vi "WriteSave2MarkdownWithImages.vi"(0 "Measurement type":T3(ring)=enum."Spectrum", 1 "Full Comment":string, 2 "Params Save":T2, 3 "Written Dataset Name":string, 4 "Log file":string caption="Status") -> (5 "Log file after":string)   [LabVIEW 2019]
uses:
  TypeDefs/AcqMode.ctl
panel:
  out "Experiment Name":string
  out "ExperimentTag":string
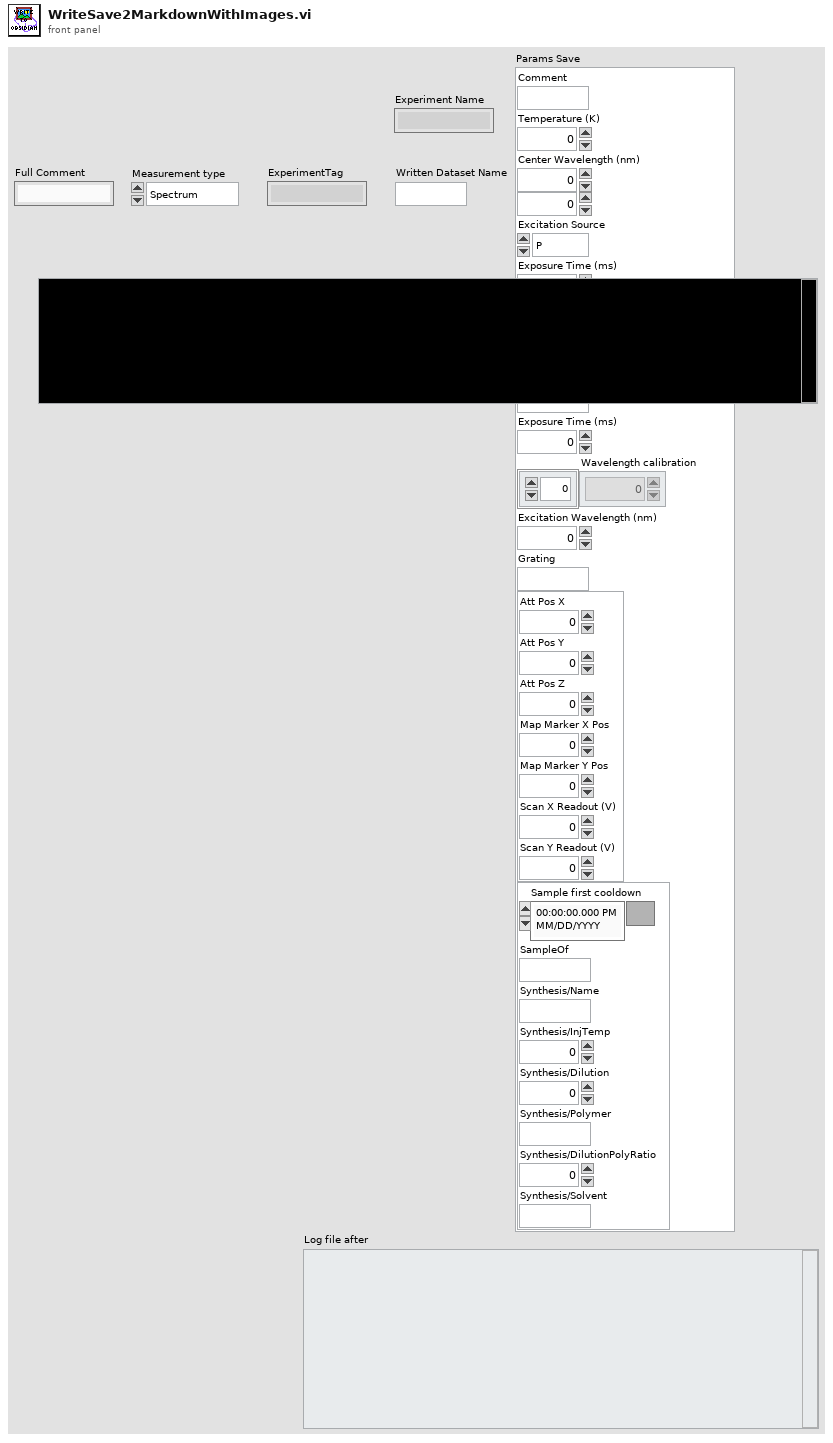
[diagram p1: front panel]
types:
  T1 = typedef "AcqMode.ctl" = enum16{"Image", "Spectrum", "APD 1", "APD 2", "APD 1+2"}
  T2 = cluster{"Comment":string, "Temperature (K)":dbl, "Center Wavelength (nm)":dbl, "Numeric":dbl, "Excitation Source":enum16{"P", "CW", "SK"}, "Exposure Time (ms)":dbl, "Experiment Name":string, "Acq Mode":T1, "Log file":string, "Exposure Time (ms)":dbl, "Wavelength calibration":dbl[], "Excitation Wavelength (nm)":dbl, "Grating":string, "Cluster":cluster{"Att Pos X":dbl, "Att Pos Y":dbl, "Att Pos Z":dbl, "Map Marker X Pos":i8, "Map Marker Y Pos":i8, "Scan X Readout (V)":dbl, "Scan Y Readout (V)":dbl}, "Cluster":cluster{"Sample first cooldown":timestamp, "SampleOf":string, "Synthesis/Name":string, "Synthesis/InjTemp":dbl, "Synthesis/Dilution":dbl, "Synthesis/Polymer":string, "Synthesis/DilutionPolyRatio":dbl, "Synthesis/Solvent":string}}
  T3 = enum16{"Time Trace", "Contrast", "XY Intensity Map", "Polarisation", "Spectrum", "Michelson", "fPow"}
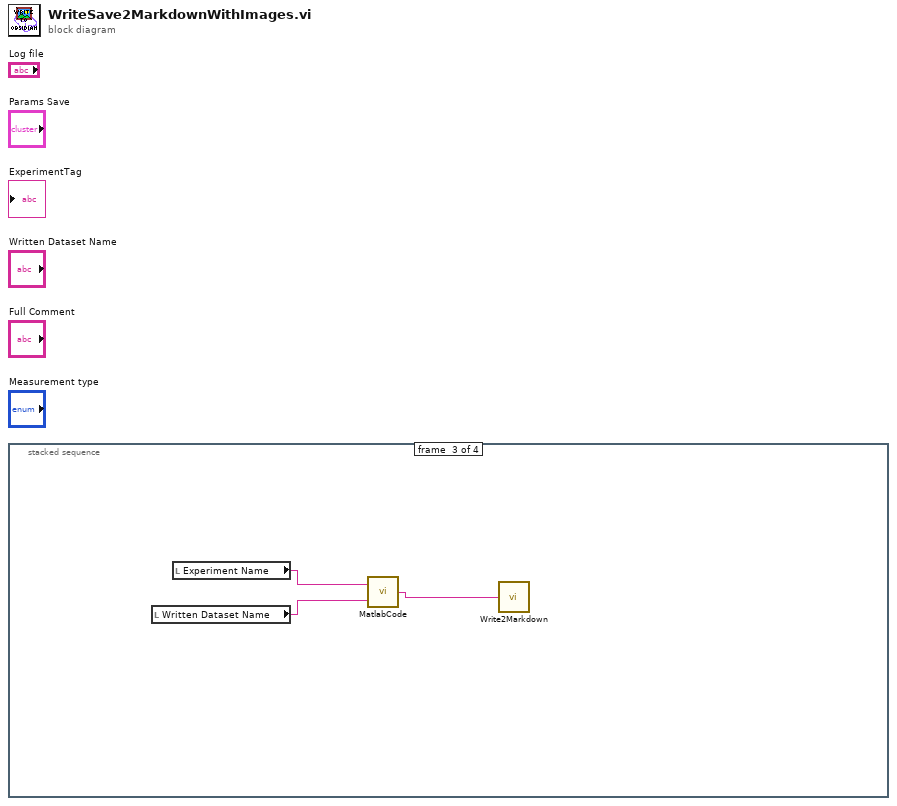
[diagram p0: block diagram]
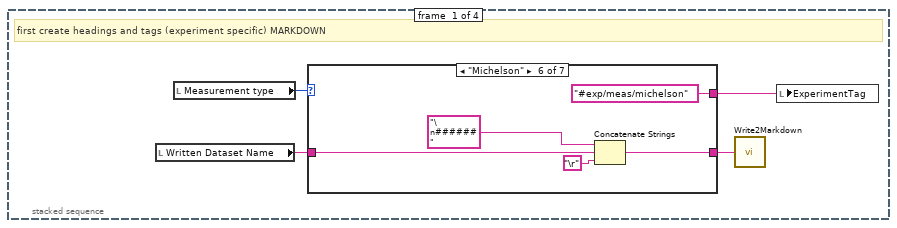
[diagram p2: hidden frame]
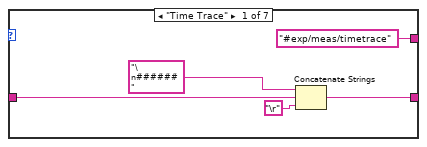
[diagram p3: hidden frame]
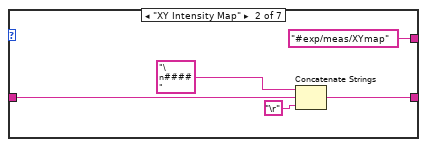
[diagram p4: hidden frame]
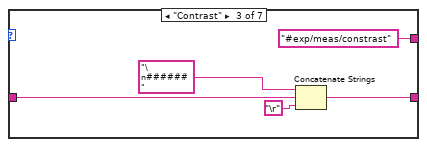
[diagram p5: hidden frame]
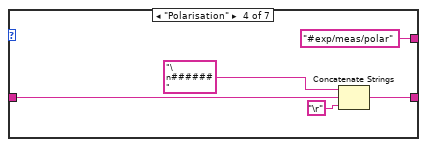
[diagram p6: hidden frame]
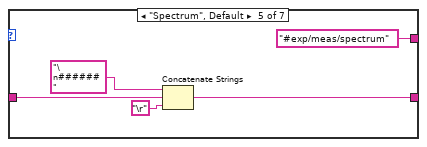
[diagram p7: hidden frame]
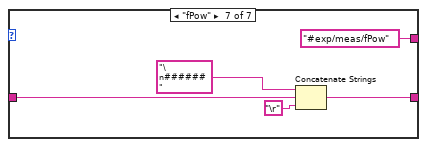
[diagram p8: hidden frame]
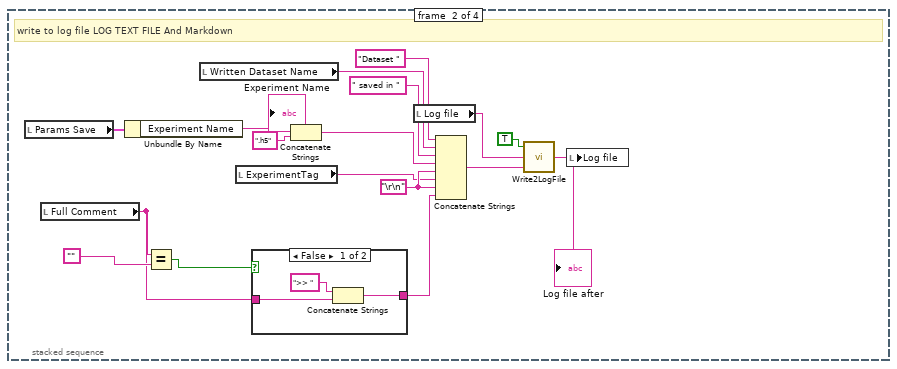
[diagram p9: hidden frame]
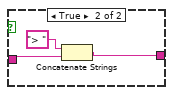
[diagram p10: hidden frame]
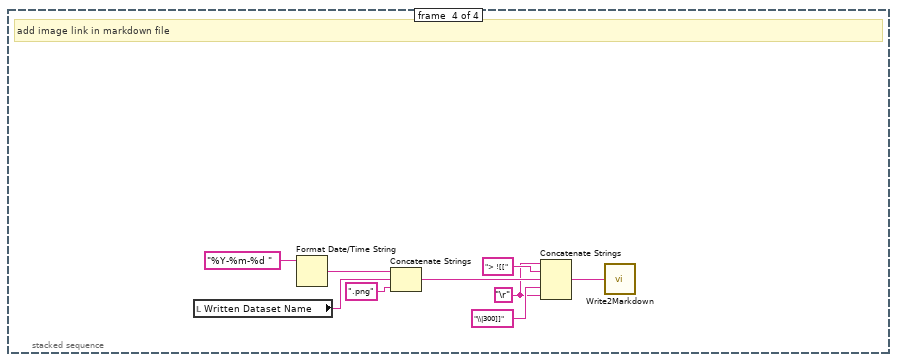
[diagram p11: hidden frame]
diagram:
  n1 = stacked-sequence {
    frame #0 {
      # "first create headings and tags (experiment specific) MARKDOWN"
      n2 = local read "Written Dataset Name"() -> (w2:string)
      n3 = local read "Measurement type"() -> (w3:T3)
      n4 = case shown="\"Michelson\"" w3 {
        tunnel: ["#exp/meas/timetrace" "#exp/meas/XYmap" "#exp/meas/constrast" "#exp/meas/polar" "#exp/meas/spectrum" "#exp/meas/michelson" "#exp/meas/fPow"] -> w1
        tunnel: [w5 w11 w15 w20 w26 w30 w35] -> w4
        tunnel: w2 -> [w7 w12 w17 w22 w25 w32 w37]
        frame "Time Trace" {
          n5 = Concatenate Strings("\n######  ", w7, "\r") -> (w5:string)
        }
        frame "XY Intensity Map" {
          n6 = Concatenate Strings("\n#### ", w12, "\r") -> (w11:string)
        }
        frame "Contrast" {
          n7 = Concatenate Strings("\n######  ", w17, "\r") -> (w15:string)
        }
        frame "Polarisation" {
          n8 = Concatenate Strings("\n###### ", w22, "\r") -> (w20:string)
        }
        frame "Spectrum", Default {
          n9 = Concatenate Strings("\n######  ", w25, "\r") -> (w26:string)
        }
        frame "Michelson" {
          n10 = Concatenate Strings("\n###### ", w32, "\r") -> (w30:string)
        }
        frame "fPow" {
          n11 = Concatenate Strings("\n######  ", w37, "\r") -> (w35:string)
        }
      }
      n12 = call "Write2Markdown.vi"("String"=w4) -> ()
      n13 = local write "ExperimentTag"(w1) -> ()
    }
    frame #1 {
      w49 = "\r\n"
      # "write to log file LOG TEXT FILE And Markdown"
      n14 = local read "Params Save"() -> (w53:T2)
      n15 = local read "Full Comment"() -> (w42:string)
      n16 = Unbundle By Name(w53) -> ("Experiment Name"=w52:string)
      "Experiment Name" <- w52
      n17 = Equal?(x=w42, y="") -> (x = y?=w43:bool)
      n18 = local read "Written Dataset Name"() -> (w55:string)
      n19 = local read "ExperimentTag"() -> (w48:string)
      n20 = case shown="False" w43 {
        tunnel: w42 -> [w58 w61]
        tunnel: [w57 w60] -> w41
        frame False {
          n21 = Concatenate Strings(">> " ("string"), w58) -> (w57:string)
        }
        frame True {
          n22 = Concatenate Strings("> " ("string"), w61) -> (w60:string)
        }
      }
      n23 = Concatenate Strings(w52, ".h5") -> (w50:string)
      n24 = local read "Log file"() -> (w46:string)
      n25 = Concatenate Strings("Dataset " ("string"), w55, " saved in " ("string"), w50, w49, w48, w49, w41) -> (w40:string)
      n26 = call "Write2LogFile.vi"("Add to log file"=w40, "Log file before"=w46, "Checkbox"=TRUE) -> ("Log file after"=w45:string)
      "Log file after" <- w45
      n27 = local write "Log file"(w45) -> ()
    }
    frame #2 {
      n28 = local read "Written Dataset Name"() -> (w63:string)
      n29 = local read "Experiment Name"() -> (w64:string)
      n30 = call "MatlabCode.vi"("Writtendatasetname"=w63, "Datasetname"=w64) -> ("concatenated string"=w65:string)
      n31 = call "Write2Markdown.vi"("String"=w65) -> ()
    }
    frame #3 {
      w67 = "\r"
      # "add image link in markdown file"
      n32 = local read "Written Dataset Name"() -> (w71:string)
      n33 = Format Date/Time String(time format string (%c)="%Y-%m-%d ") -> (date/time string=w72:string)  [unwired: 2 in]
      n34 = Concatenate Strings(w72, w71, ".png" ("string")) -> (w70:string)
      n35 = Concatenate Strings(w67, "> ![[", w70, "\\|300]]", w67) -> (w66:string)
      n36 = call "Write2Markdown.vi"("String"=w66) -> ()
    }
  }
